vi "Reinitialize.vi"(8 "error in (no error)":errorcluster, 11 "Comdel in":refnum<class "PL Comdel CX.lvclass">) -> (0 "error out":errorcluster, 3 "Comdel out":refnum<class "PL Comdel CX.lvclass">)   [LabVIEW 2015, in "PL Comdel CX.lvclass"]
doc: "Reinitializes connection to device based on previously specified settings."
uses:
  PL Comdel CX.lvclass
  PL Comdel CX.lvclass/PL Comdel CX.ctl
  <vilib>/Instr/_visa.llb/VISA Configure Serial Port (Instr).vi
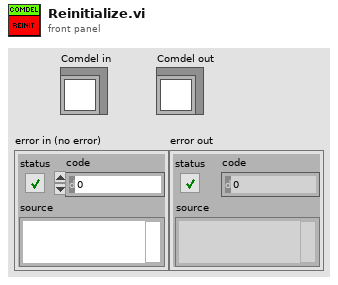
[diagram p1: front panel]
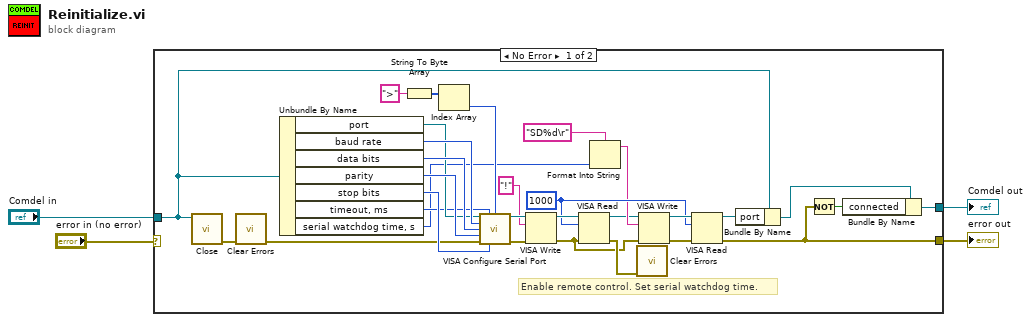
[diagram p0: block diagram]
diagram:
  n1 = case shown="No Error" "error in (no error)" {
    selector: "error in (no error)" -> [_ w35]
    tunnel: "Comdel in" -> [w34 w36]
    tunnel: [w31 w36] -> w3
    tunnel: [w14 w35] -> w2
    frame No Error {
      w12 = u32 1000 ("byte count")
      # "Enable remote control. Set serial watchdog time."
      n2 = call "Close.vi"("Comdel in"=w34) -> ("error out"=w6:errorcluster)  [unwired: 10 in]
      n3 = call <vilib>:"Clear Errors.vi"("error in (no error)"=w6) -> ("error out"=w5:errorcluster)  [unwired: 5 in, 1 out]
      n4 = Unbundle By Name(w34) -> ("port"=w26:refnum<visa-resource-name>, "baud rate"=w30:u32, "data bits"=w29:u16, "parity"=w28:u16, "stop bits"=w27:u16, "timeout, ms"=w8:u32, "serial watchdog time, s"=w7:u16)
      n5 = String To Byte Array(string=">") -> (unsigned byte array=w24:u8[])
      n6 = Index Array(array=w24) -> (element=w23:u8)  [unwired: 1 in]
      n7 = call-poly "VISA Configure Serial Port"("VISA resource name"=w26, "timeout (10sec)"=w8, "termination char\n(0xA = '\\n' = LF)"=w23, "baud rate (9600)"=w30, "data bits (8)"=w29, "parity (0:none)"=w28, "error in (no error)"=w5, "stop bits (10: 1 bit)"=w27) -> ("VISA resource name out"=w22:refnum<visa-resource-name>, "error out"=w21:errorcluster)  [unwired: 6 in]
      n8 = VISA Write(VISA resource name=w22, write buffer="!", error in (no error)=w21) -> (VISA resource name out=w19:refnum<visa-resource-name>, error out=w10:errorcluster)  [unwired: 1 out]
      n9 = VISA Read(VISA resource name=w19, byte count=w12, error in (no error)=w10) -> (VISA resource name out=w9:refnum<visa-resource-name>, error out=w17:errorcluster)  [unwired: 2 out]
      n10 = Format Into String(format string="SD%d\r", w7) -> (resulting string=w11:string)  [unwired: 2 in, 1 out]
      n11 = call <vilib>:"Clear Errors.vi"("error in (no error)"=w17) -> ()  [unwired: 5 in, 2 out]
      n12 = VISA Write(VISA resource name=w9, write buffer=w11, error in (no error)=w10) -> (VISA resource name out=w16:refnum<visa-resource-name>, error out=w15:errorcluster)  [unwired: 1 out]
      n13 = VISA Read(VISA resource name=w16, byte count=w12, error in (no error)=w15) -> (VISA resource name out=w13:refnum<visa-resource-name>, error out=w14:errorcluster)  [unwired: 2 out]
      n14 = Bundle By Name(cluster=w34, "port"=w13) -> (w33:refnum<class "PL Comdel CX.lvclass">)
      n15 = Not(x=w14) -> (.not. x?=w32:bool)
      n16 = Bundle By Name(cluster=w33, "connected"=w32) -> (w31:refnum<class "PL Comdel CX.lvclass">)
    }
    frame Error {
    }
  }
  "Comdel out" <- w3
  "error out" <- w2
